vi "Controller Process.vi"(8 "error in (no error)":errorcluster, 11 "View Model":T1) -> (0 "error out":errorcluster)   [LabVIEW 2017]
doc: "A SW component that monitors and controls the Elevator movement by interacting with other processes."
uses:
  View Model/Controls/View Model.ctl
  View Model/Controls/Shared Model.ctl
  Error/Controls/Error Model.ctl
  Error/Controls/Error Event.ctl
  Error/Controls/Error Type.ctl
  Configuration/Controls/Config DB Model.ctl
  Configuration/Controls/Config DB Command.ctl
  Configuration/Controls/Config DB Record.ctl
  Controls/Controller Model.ctl
  Controls/Elevator Location.ctl
  Controls/Elevator Direction Event.ctl
  Controls/Elevator Direction.ctl
  Controls/Elevator CMD Event.ctl
  Controls/Elevator Commands.ctl
  Controls/Elevator Overhead.ctl
  Controls/Elevator State.ctl
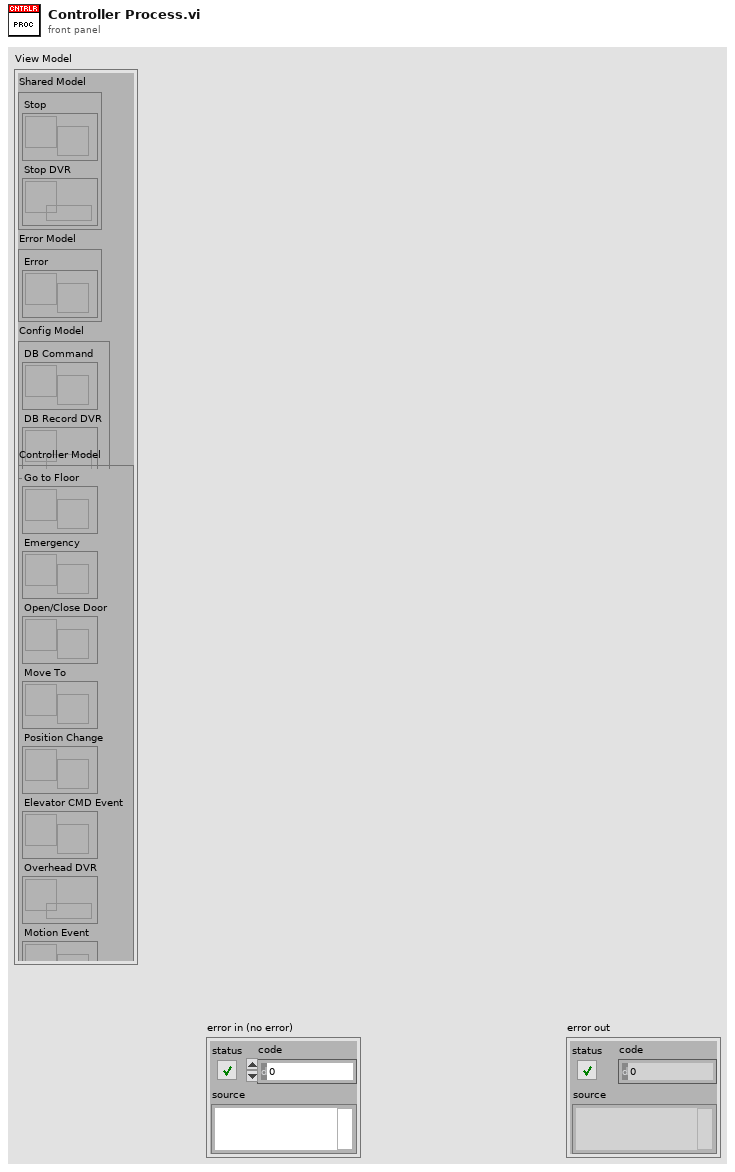
[diagram p1: front panel]
types:
  T1 = typedef "View Model.ctl" = cluster{"Shared Model":T2, "Error Model":T3, "Config Model":T4, "Controller Model":T5}
  T2 = typedef "Shared Model.ctl" = cluster{"Stop":refnum<user-event>, "Stop DVR":refnum<data-value>}
  T3 = typedef "Error Model.ctl" = cluster{"Error":refnum<user-event>}
  T4 = typedef "Config DB Model.ctl" = cluster{"DB Command":refnum<user-event>, "DB Record DVR":refnum<data-value>}
  T5 = typedef "Controller Model.ctl" = cluster{"Go to Floor":refnum<user-event>, "Emergency":refnum<user-event>, "Open/Close Door":refnum<user-event>, "Move To":refnum<user-event>, "Position Change":refnum<user-event>, "Elevator CMD Event":refnum<user-event>, "Overhead DVR":refnum<data-value>, "Motion Event":refnum<user-event>}
  T6 = typedef "Elevator Location.ctl" = enum16{"1st Floor", "2nd Floor", "3rd Floor", "4th Floor"}
  T7 = typedef "Elevator Commands.ctl" = enum16{"Go Up", "Go Down", "Go to Floor", "Emergency", "Open Doors", "Close Doors"}
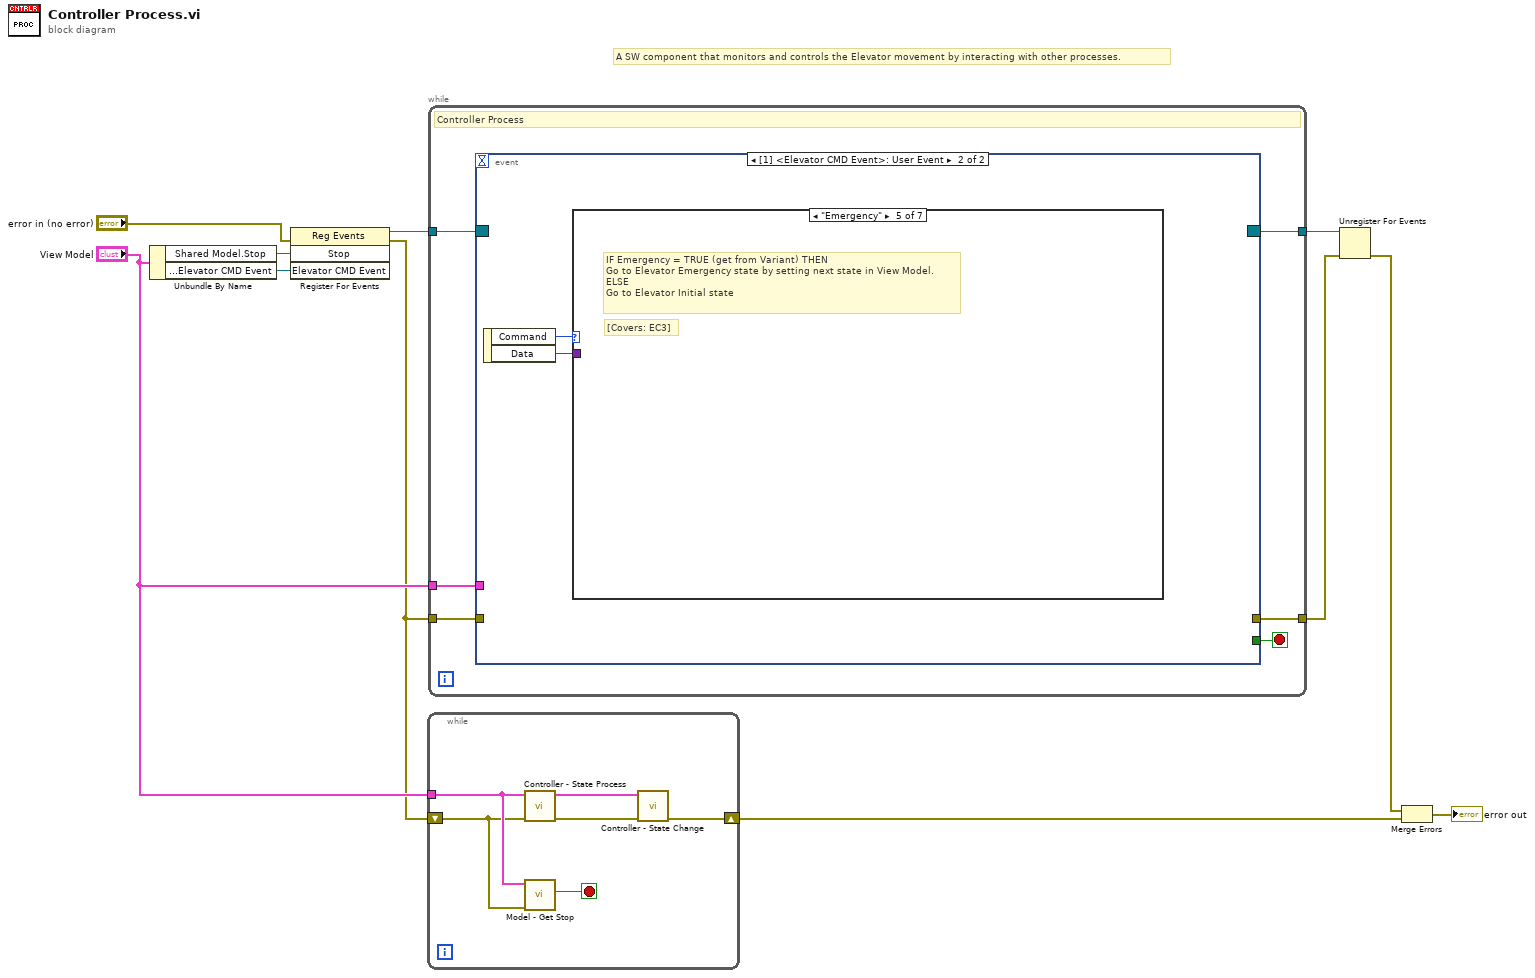
[diagram p0: block diagram]
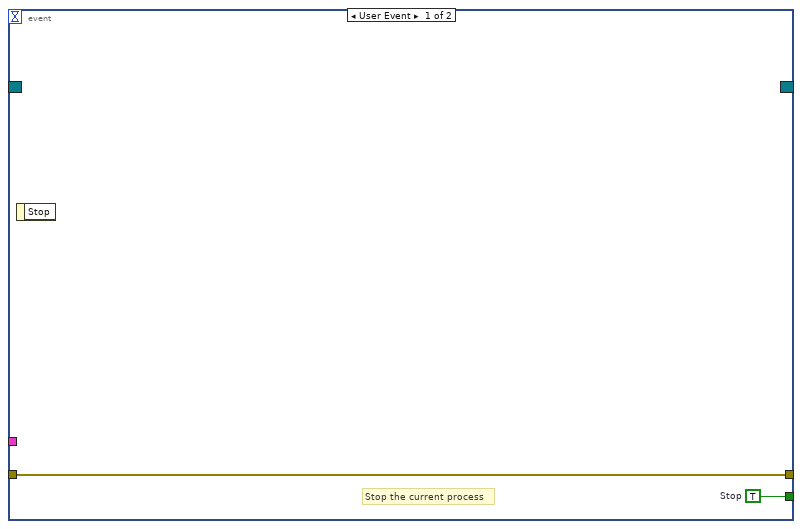
[diagram p2: hidden frame]
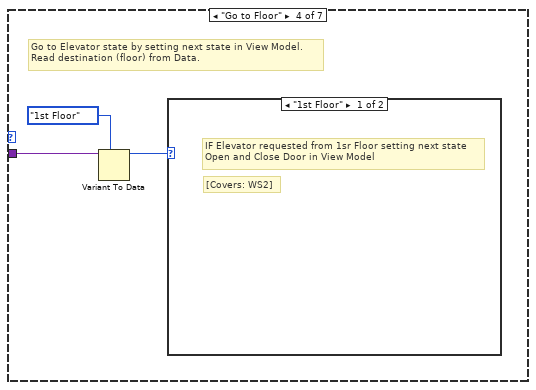
[diagram p6: hidden frame]
diagram:
  # "A SW component that monitors and controls the Elevator movement by interacting with other processes."
  n1 = Unbundle By Name("View Model") -> ("Shared Model.Stop"=w11:refnum<user-event>, "Controller Model.Elevator CMD Event"=w1:refnum<user-event>)
  n2 = register-events(error in="error in (no error)", w11, w1) -> (reference out=w10:refnum<event-registration>, error out=w5:errorcluster)  [unwired: 1 in]
  n3 = while {
    tunnel: "View Model" -> [w15]
    shift-right: [w12] -> w4
    shift-left: w5 -> [w14]
    stop <- w13 stop-if-true
    n4 = call "Controller - State Process.vi"("error in (no error)"=w14, "View Model"=w15) -> ("error out"=w17:errorcluster, "View Model"=w16:T1)  [unwired: 8 in]
    n5 = call "Model - Get Stop.vi"("error in (no error)"=w14, "View Model"=w15) -> ("Stop?"=w13:bool)  [unwired: 7 in, 2 out]
    n6 = call "Controller - State Change.vi"("error in (no error)"=w17, "View Model"=w16) -> ("error out"=w12:errorcluster)  [unwired: 8 in, 1 out]
  }
  n7 = while {
    tunnel: w10 -> [w23]
    tunnel: [w22] -> w9
    tunnel: w5 -> [w21]
    tunnel: "View Model" -> [w20]
    tunnel: [w19] -> w7
    stop <- w18 stop-if-true
    # "Controller Process"
    n8 = event shown="[1] <Elevator CMD Event>: User Event" {
      selector: w23 -> [_ _]
      dyn-events: [_ _] -> w22
      timeout: _ -> [_ _]
      tunnel: w21 -> [w25 _]
      tunnel: w20 -> [_ _]
      tunnel: [w25 _] -> w19
      tunnel: [w24 _] -> w18
      event User Event {
        w24 = TRUE  # Stop
        # "Stop the current process"
        n9 = event-data() -> ()  [unwired: 1 in, 1 out]
      }
      event User Event {
        n10 = event-data() -> ("Command"=w27:T7, "Data"=w26:variant)  [unwired: 1 in]
        n11 = case shown="\"Emergency\"" w27 {
          tunnel: w26 -> [_ _ _ w30 _ _ _]
          frame Default {
          }
          frame "Go Up" {
            # "Go to Elevator Start and Move state by setting next state in View Model.\nSet movement direction = Up\nRead departure from Data"
          }
          frame "Go Down" {
            # "Go to Elevator Start and Move state by setting next state in View Model.\nSet movement direction = Down\nRead departure from Data"
          }
          frame "Go to Floor" {
            # "Go to Elevator state by setting next state in View Model.\nRead destination (floor) from Data."
            n12 = Variant To Data(type=Elevator_Location."1st Floor" ("Destination"), Variant=w30) -> (data=w28:T6)  [unwired: 1 in, 1 out]
            n13 = case shown="\"1st Floor\"" w28 {
              frame "1st Floor" {
                # "[Covers: WS2]"
                # "IF Elevator requested from 1sr Floor setting next state\nOpen and Close Door in View Model"
              }
              frame Default {
                # "[Covers: WS3]"
                # "IF Elevator requested NOT from 1sr Floor \nsetting next state Continue Travel in View Model"
              }
            }
          }
          frame "Emergency" {
            # "[Covers: EC3]"
            # "IF Emergency = TRUE (get from Variant) THEN\nGo to Elevator Emergency state by setting next state in View Model.\nELSE\nGo to Elevator Initial state"
          }
          frame "Open Doors" {
            # "Go to Elevator Open/Close Door state by setting next state in View Model."
          }
          frame "Close Doors" {
            # "Go to Elevator Open/Close Door state by setting next state in View Model."
          }
        }
      }
    }
  }
  n14 = Unregister For Events(event registration refnum=w9, error in=w7) -> (error out=w3:errorcluster)
  n15 = Merge Errors(w3, w4) -> (→"error out":errorcluster)
